vi "PDP MagStatus= Message.vi"(0 "Mag Status":i32(ring) items=["Hold", "To Setpoint", "To Zero"]) -> ()   [LabVIEW 2019]
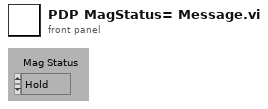
[diagram p1: front panel]
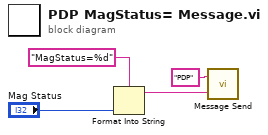
[diagram p0: block diagram]
diagram:
  n1 = Format Into String(format string="MagStatus=%d" ("Format String"), "Mag Status") -> (resulting string=w1:string)  [unwired: 2 in, 1 out]
  n2 = call "Message Send.vi"("Message"=w1, "Destination"="PDP") -> ()
